vi "LV to gRPC Timestamp.vi"(11 "LV Timestamp":timestamp) -> (3 "gRPC Timestamp":T1)   [LabVIEW 2023, in "Head Worker.lvclass"]
doc: "Convert LabVIEW timestamp data to gRPC timestamp data."
uses:
  Head Worker.lvclass
  Generated_server/RPC Messages/google_protobuf_Timestamp.ctl
  <vilib>/LabVIEW Open Source Project/Epoch Date & Time/epoch.UNIX/Epoch.UNIX.lvclass
  C:/Program Files (x86)/National Instruments/LabVIEW 2023/vi.lib/LabVIEW Open Source Project/Epoch Date & Time/epoch/Epoch.lvclass
  <vilib>/LabVIEW Open Source Project/Epoch Date & Time/Get Epoch Time.vi
  Head Worker.lvclass/Head Worker.ctl
  Generated_server/Generated_server.lvlib
panel:
  # "Connector Pane"
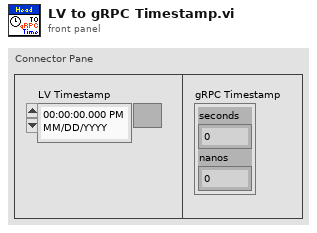
[diagram p1: front panel]
types:
  T1 = typedef "Generated_server.lvlib/google_protobuf_Timestamp.ctl" = cluster{"seconds":i64, "nanos":i32}
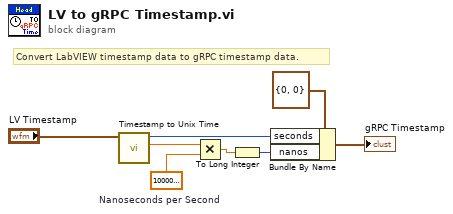
[diagram p0: block diagram]
diagram:
  w7 = 1000000000.0  # Nanoseconds per Second
  # "Convert LabVIEW timestamp data to gRPC timestamp data."
  n1 = call <vilib>:"Timestamp to Unix Time.vi"("Timestamp (now)"="LV Timestamp") -> ("Fractional Second"=w4:dbl, "Unix Time (s)"=w5:i64)  [unwired: 9 in]
  n2 = Multiply(x=w4, y=w7) -> (x*y=w6:dbl)
  n3 = To Long Integer(number=w6) -> (32bit integer=w3:i32)
  n4 = Bundle By Name(cluster=T1 {"seconds"=0, "nanos"=0} ("t0"), "seconds"=w5, "nanos"=w3) -> (→"gRPC Timestamp":T1)
